vi "Test Labels.vi"() -> ()   [LabVIEW 2020]
uses:
  src/metrics/counter/Counter.lvclass
  src/registry/session/Registry Session.lvclass
  src/metrics/gauge/Gauge.lvclass
  src/metrics/histogram/Histogram.lvclass
panel:
  in  "Channel":string(combo)
  in  "Board":string(combo)
  out "Metric Names":string[](array[string])
  out "Next Timeout":i32
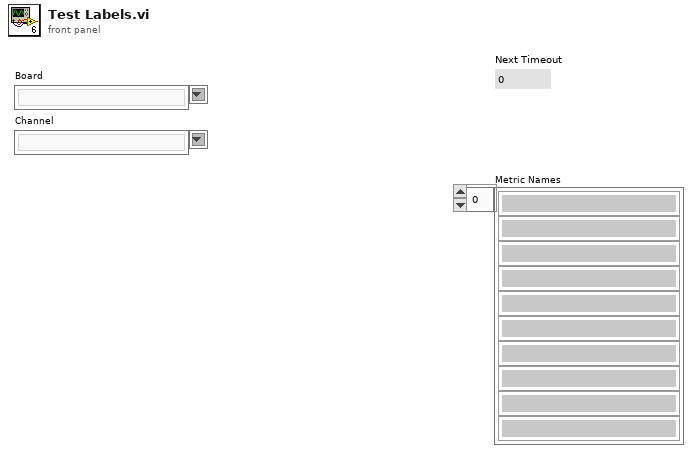
[diagram p1: front panel]
types:
  T1 = typedef "Registry.lvlib/Registry Session.lvclass/Session Handle.ctl" = refnum<data-value>
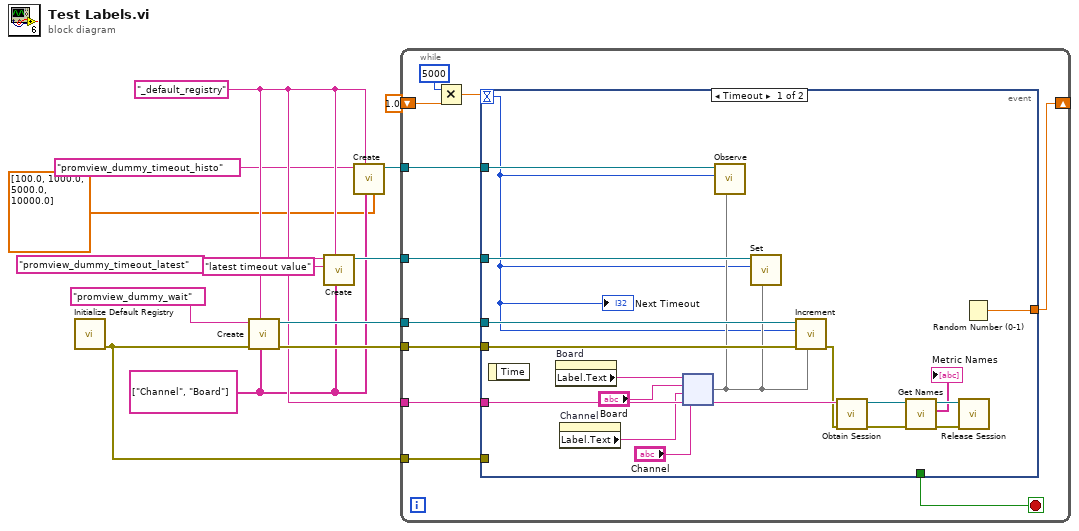
[diagram p0: block diagram]
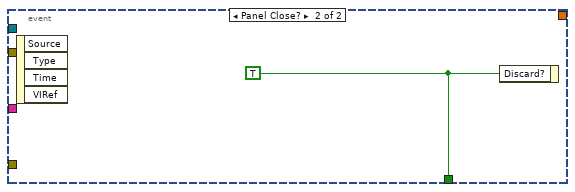
[diagram p2: hidden frame]
diagram:
  w3 = string[] ["Channel", "Board"] ("Label Names")
  w4 = "_default_registry" ("Registry Name")
  n1 = call "Initialize Default Registry.vi"() -> ("error out"=w10:errorcluster)  [unwired: 9 in, 2 out]
  n2 = call "Create.vi"("Label Names"=w3, "Registry Name"=w4, "error in (no error)"=w10, "Metric Name"="promview_dummy_wait") -> ("error out"=w9:errorcluster, "Counter Ref"=w13:refnum<data-value>)  [unwired: 6 in]
  n3 = call "Create.vi"("Label Names"=w3, "Registry Name"=w4, "Description"="latest timeout value", "Metric Name"="promview_dummy_timeout_latest") -> ("Gauge Ref"=w6:refnum<data-value>)  [unwired: 6 in, 1 out]
  n4 = call "Create.vi"("Buckets"=dbl[] [100.0, 1000.0, 5000.0, 10000.0], "Label Names"=w3, "Registry Name"=w4, "Name"="promview_dummy_timeout_histo") -> ("Histogram Ref"=w5:refnum<data-value>)  [unwired: 6 in, 1 out]
  n5 = while {
    tunnel: w13 -> [w23]
    tunnel: w4 -> [w22]
    shift-right: [w20] -> _
    shift-left: 1.0 ("number: 0 to 1") -> [w19]
    tunnel: w10 -> [w17]
    tunnel: w9 -> [w16]
    tunnel: w6 -> [w15]
    tunnel: w5 -> [w14]
    stop <- w24 stop-if-true
    n6 = Multiply(x=5000, y=w19) -> (x*y=w18:dbl)
    n7 = event shown="[0] Timeout" {
      selector: _ -> [_ _]
      dyn-events: _ -> [_ _]
      timeout: w18 -> [w25 _]
      tunnel: [_ w43] -> w24
      tunnel: w23 -> [w42 _]
      tunnel: w22 -> [w41 _]
      tunnel: [w36 _] -> w20
      tunnel: w17 -> [_ _]
      tunnel: w16 -> [w35 _]
      tunnel: w15 -> [w28 _]
      tunnel: w14 -> [w27 _]
      event Timeout {
        n8 = event-data() -> ()  [unwired: 1 in, 1 out]
        n9 = property on="Board" class="CmbBox"() -> ("Label.Text"=w29:string)  [unwired: 2 in, 2 out]
        n10 = property on="Channel" class="CmbBox"() -> ("Label.Text"=w31:string)  [unwired: 2 in, 2 out]
        n11 = node(w29, "Board", w31, "Channel") -> (w26:map{string, string})
        n12 = call "Observe.vi"("Labels"=w26, "New Value"=w25, "Histogram Ref"=w27) -> ()  [unwired: 7 in, 2 out]
        n13 = call "Set.vi"("Labels"=w26, "Value"=w25, "Gauge Ref"=w28) -> ()  [unwired: 7 in, 2 out]
        n14 = call "Increment.vi"("Labels"=w26, "error in (no error)"=w35, "Step"=w25, "Counter Ref"=w42) -> ("error out"=w40:errorcluster)  [unwired: 6 in, 1 out]
        n15 = call "Obtain Session.vi"("error in (no error)"=w40, "Session  Name ()"=w41) -> ("error out"=w34:errorcluster, "Session Handle"=w37:T1)  [unwired: 8 in]
        n16 = call "Get Names.vi"("error in (no error)"=w34, "Session Handle in"=w37) -> ("error out"=w33:errorcluster, "Metric Names"=→"Metric Names":string[], "Session Handle out"=w39:T1)  [unwired: 7 in]
        n17 = call "Release Session.vi"("error in (no error)"=w33, "Session Handle"=w39) -> ()  [unwired: 9 in, 1 out]
        n18 = Random Number (0-1)() -> (number: 0 to 1=w36:dbl)
        "Next Timeout" <- w25
      }
      event Panel Close? {
        w43 = TRUE ("Discard?")
        n19 = event-data() -> ()  [unwired: 1 in, 4 out]
        n20 = event-data("Discard?"=w43) -> ()  [unwired: 1 in, 1 out]
      }
    }
  }
